vi "Pre Launch Init.vi"(11 "CI Mediator in":refnum<class "CI Mediator.lvclass">) -> (0 "error out":errorcluster, 3 "CI Mediator out":refnum<class "CI Mediator.lvclass">)   [LabVIEW 2014, in "CI Mediator.lvlib" / "CI Mediator.lvclass"]
doc: "(<B>Filename</B>: Actor Framework.lvlib:Actor.lvclass:Pre Launch Init.vi)\n\nDefines behavior that occurs after the Launch Nested Actor method is invoked but before the actor's Actor Core method begins running.\n\nBy default, this method does nothing. A descendant class may override it to define behavior."
uses:
  CI Mediator.lvclass
  <vilib>/ActorFramework/Actor/Actor.lvclass/Actor.ctl
  <vilib>/ActorFramework/Message Enqueuer/Message Enqueuer.lvclass/Message Enqueuer.ctl
  CI Mediator.lvclass/CI Mediator.ctl
  Controls/Executor Status - STYP.ctl
  <vilib>/ActorFramework/Message Enqueuer/Init from Existing Queue.vi
  <vilib>/ActorFramework/Message Enqueuer/Message Enqueuer.lvclass
  <vilib>/ActorFramework/Actor/Actor.lvclass
  Classes/Executor/Executor.lvclass
  Classes/Log File/Log File.lvclass
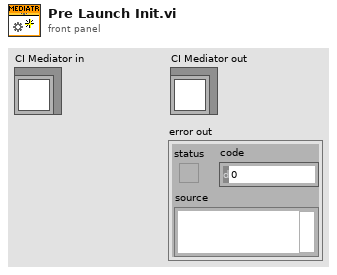
[diagram p1: front panel]
types:
  T1 = typedef "Executor Status - STYP.ctl" = cluster{"Executor Name":string, "Status":bool}
  T2 = cluster{"Stop":refnum<user-event>, "Executor Status":refnum<user-event>}
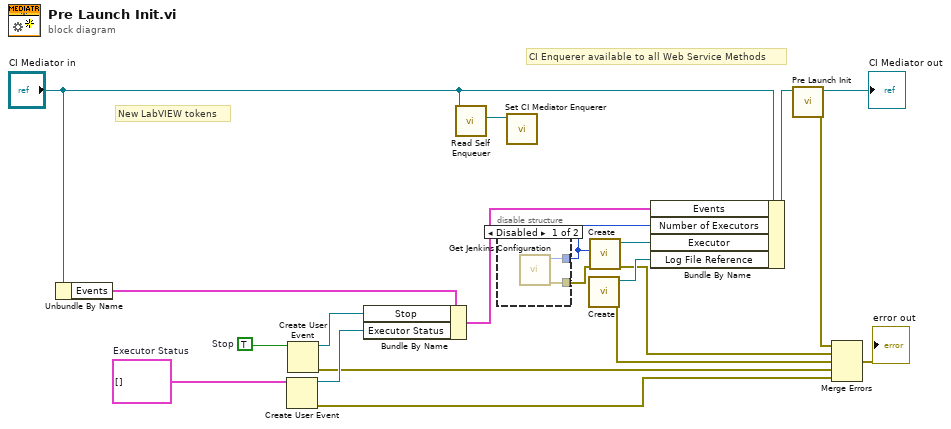
[diagram p0: block diagram]
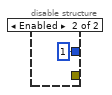
[diagram p2: hidden frame]
diagram:
  w15 = TRUE  # Stop
  w16 = T1[] []  # Executor Status
  # "New LabVIEW tokens"
  # "CI Enquerer available to all Web Service Methods"
  n1 = Unbundle By Name("CI Mediator in") -> ("Events"=w12:T2)
  n2 = Create User Event(user event datatype=w16) -> (user event=w13:refnum<user-event>, error out=w4:errorcluster)  [unwired: 1 in]
  n3 = Create User Event(user event datatype=w15) -> (user event=w14:refnum<user-event>, error out=w5:errorcluster)  [unwired: 1 in]
  n4 = Bundle By Name(cluster=w12, "Stop"=w14, "Executor Status"=w13) -> (w11:T2)
  n5 = call <vilib>:"Read Self Enqueuer.vi"("Actor"="CI Mediator in") -> ("Self Enqueuer"=w1:refnum<class "Message Enqueuer.lvclass">)  [unwired: 10 in]
  n6 = disable-structure shown="Disabled" {
    disable-tunnel: [w22 1 ("Number of Executors")] -> w3
    disable-tunnel: [w21 _] -> w8
    frame Disabled {
      n7 = call "Get Jenkins Configuration.vi"() -> ("error out"=w21:errorcluster, "Number of Executors"=w22:i32)  [unwired: 10 in]
    }
    frame Enabled {
    }
  }
  n8 = call "Set CI Mediator Enquerer.vi"("Actor's Enqueuer"=w1) -> ()  [unwired: 10 in, 1 out]
  n9 = call "Create.vi"() -> ("error out"=w6:errorcluster, "Log File Ref"=w9:refnum<data-value>)  [unwired: 10 in]
  n10 = call "Create.vi"("error in (no error)"=w8, "Number of Executors"=w3) -> ("error out"=w7:errorcluster, "Executor"=w10:refnum<class "Executor.lvclass">)  [unwired: 8 in]
  n11 = Bundle By Name(cluster="CI Mediator in", "Events"=w11, "Number of Executors"=w3, "Executor"=w10, "Log File Reference"=w9) -> (w18:refnum<class "CI Mediator.lvclass">)
  n12 = call-parent "Pre Launch Init.vi"("Actor in"=w18) -> ("error out"=w19:errorcluster, "Actor out"=→"CI Mediator out":refnum<class "CI Mediator.lvclass">)  [unwired: 9 in]
  n13 = Merge Errors(w19, w7, w6, w5, w4) -> (→"error out":errorcluster)
